vi "get_settings_cluster.vi"(8 "error in (no error)":errorcluster, 11 "ScanModeTS090821Circular2D in":refnum<class "ImagingModeTS090821Circular2D.lvclass">) -> (0 "error out":errorcluster, 2 "settings cluster":variant, 3 "ScanModeTS090821Circular2D out":refnum<class "ImagingModeTS090821Circular2D.lvclass">)   [LabVIEW 2010, in "ImagingModeTS090821Circular2D.lvclass"]
uses:
  ImagingModeTS090821Circular2D.lvclass
  ImagingModeTS090821Circular2D.lvclass/ImagingModeTS090821Circular2D.ctl
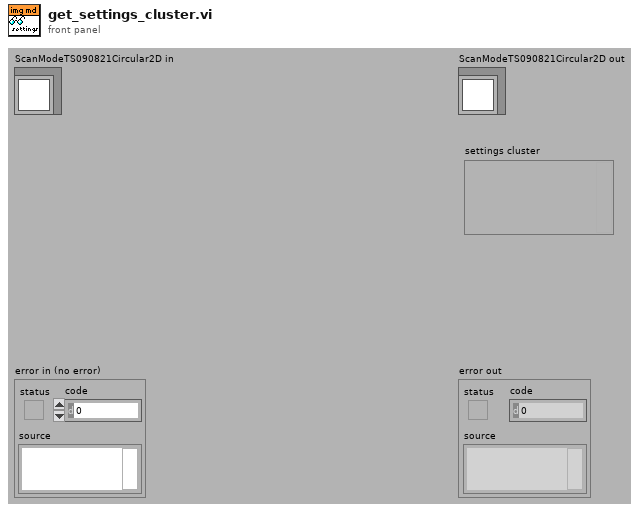
[diagram p1: front panel]
types:
  T1 = typedef "ImagingModeTS090821Circular2D.lvclass/settings_cluster.ctl" = cluster{"AmplitudeX":dbl[unit], "AmplitudeY":dbl[unit], "FrequencyY":dbl, "FrequencyX":dbl, "PhaseShift":dbl, "CenterX":dbl, "CenterY":dbl, "RotationAngle":dbl, "ScanRate":dbl[unit], "Spiral":bool, "DumpFactor":dbl, "TotalPixelsPerCycle":i32, "NumberOfCycles":i32, "LinesPerFrame":i32, "Double":bool}
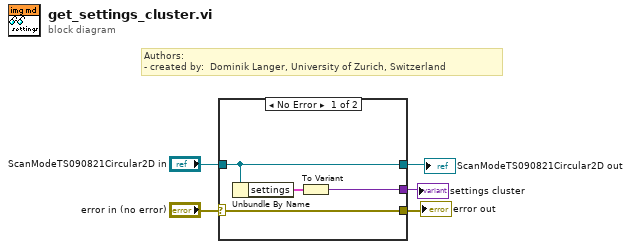
[diagram p0: block diagram]
diagram:
  # "Authors: \n- created by:  Dominik Langer, University of Zurich, Switzerland"
  n1 = case shown="No Error" "error in (no error)" {
    selector: "error in (no error)" -> [w7 w11]
    tunnel: "ScanModeTS090821Circular2D in" -> [w6 w10]
    tunnel: [w8 _] -> w3
    tunnel: [w7 w11] -> w2
    tunnel: [w6 w10] -> w1
    frame No Error {
      n2 = Unbundle By Name(w6) -> ("settings"=w9:T1)
      n3 = To Variant(anything=w9) -> (Variant=w8:variant)
    }
    frame Error {
    }
  }
  "error out" <- w2
  "ScanModeTS090821Circular2D out" <- w1
  "settings cluster" <- w3
